vi "Item_Interface.vi"() -> (3 "InterfaceTable":T1)   [LabVIEW 2020, in "Message Rescripter.lvlib"]
uses:
  Message Rescripter.lvlib
  <resource>/Framework/Providers/API/Item_Interface.ctl
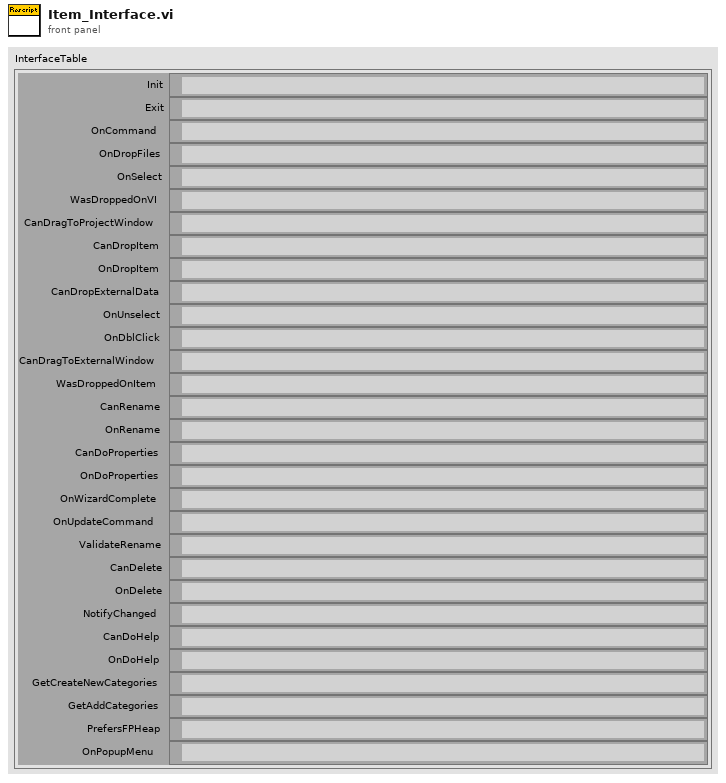
[diagram p1: front panel]
types:
  T1 = typedef "Item_Interface.ctl" = cluster{"Init":path, "Exit":path, "OnCommand":path, "OnDropFiles":path, "OnSelect":path, "WasDroppedOnVI":path, "CanDragToProjectWindow":path, "CanDropItem":path, "OnDropItem":path, "CanDropExternalData":path, "OnUnselect":path, "OnDblClick":path, "CanDragToExternalWindow":path, "WasDroppedOnItem":path, "CanRename":path, "OnRename":path, "CanDoProperties":path, "OnDoProperties":path, "OnWizardComplete":path, "OnUpdateCommand":path, "ValidateRename":path, "CanDelete":path, "OnDelete":path, "NotifyChanged":path, "CanDoHelp":path, "OnDoHelp":path, "GetCreateNewCategories":path, "GetAddCategories":path, "PrefersFPHeap":path, "OnPopupMenu":path}
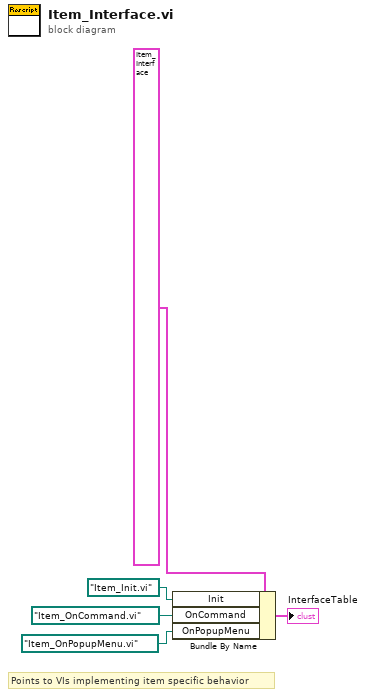
[diagram p0: block diagram]
diagram:
  # "Points to VIs implementing item specific behavior"
  n1 = Bundle By Name(cluster=T1 {"Init"=path "", "Exit"=path "", "OnCommand"=path "", "OnDropFiles"=path "", "OnSelect"=path "", "WasDroppedOnVI"=path "", "CanDragToProjectWindow"=path "", "CanDropItem"=path "", "OnDropItem"=path "", "CanDropExternalData"=path "", "OnUnselect"=path "", "OnDblClick"=path "", "CanDragToExternalWindow"=path "", "WasDroppedOnItem"=path "", "CanRename"=path "", "OnRename"=path "", "CanDoProperties"=path "", "OnDoProperties"=path "", "OnWizardComplete"=path "", "OnUpdateCommand"=path "", "ValidateRename"=path "", "CanDelete"=path "", "OnDelete"=path "", "NotifyChanged"=path "", "CanDoHelp"=path "", "OnDoHelp"=path "", "GetCreateNewCategories"=path "", "GetAddCategories"=path "", "PrefersFPHeap"=path "", "OnPopupMenu"=path ""} ("InterfaceTable"), "Init"=path "Item_Init.vi", "OnCommand"=path "Item_OnCommand.vi", "OnPopupMenu"=path "Item_OnPopupMenu.vi") -> (→"InterfaceTable":T1)
